vi "iWorx - Conductivity.vi"() -> ()   [LabVIEW 2012]
uses:
  vi.lib/iWorx/iWorx Set Points.ctl
  <vilib>/DAQmx/read.llb/DAQmx Read (Analog 1D Wfm NChan 1Samp).vi
  <vilib>/DAQmx/create/channels.llb/DAQmx Create Channel (AI-Voltage-Basic).vi
  <vilib>/DAQmx/miscellaneous.llb/DAQmx Fill In Error Info.vi
panel:
  in  "Reset Scale":bool
  in  "Stop":bool
  in  "Log Info Button":bool
  in  "Reset Default Cal":bool
  in  "Set Points":T1={"SP1 Voltage"=0.2, "SP1 Value"=20.0, "SP2 Voltage"=2.0, "SP2 Value"=200.0} {"SP2 Value" format="%.1f mS"; "SP2 Voltage" format="%.1f V"; "SP1 Value" format="%.1f mS"; "SP1 Voltage" format="%.1f V"}
  in  "Set Up":bool
  out "Offset(b)":dbl=-1.1111111111111112
  out "Slope(m)":dbl=5.277777777777778
  in  "Channel":u16(ring) items=["Channel 1", "Channel 2"]
  in  "Pause Button":bool
  in  "Snapshot":bool
  out "Processed Signal":dbl(knob) caption="Conductivity" scale=0.0..20.0
  out "Waveform Chart":waveform(dbl)(graph)
  in  "Sample Timing":u16(ring)=200 items=["20Hz"=50, "5 Hz"=200, "2 Hz"=500, "1 Hz"=1000, ".5 Hz"=2000, ".2 Hz"=5000]
  in  "Clear Chart":bool
  in  "Open Log":bool
  in  "Autoscale Y":bool
  out "Raw Signal":dbl(knob) scale=-10.0..10.0
  # "iWorx - Conductivity Probe - Data Logger"
  # "Sensor Input"
  # "(              ,              )"
  # "(              ,              )"
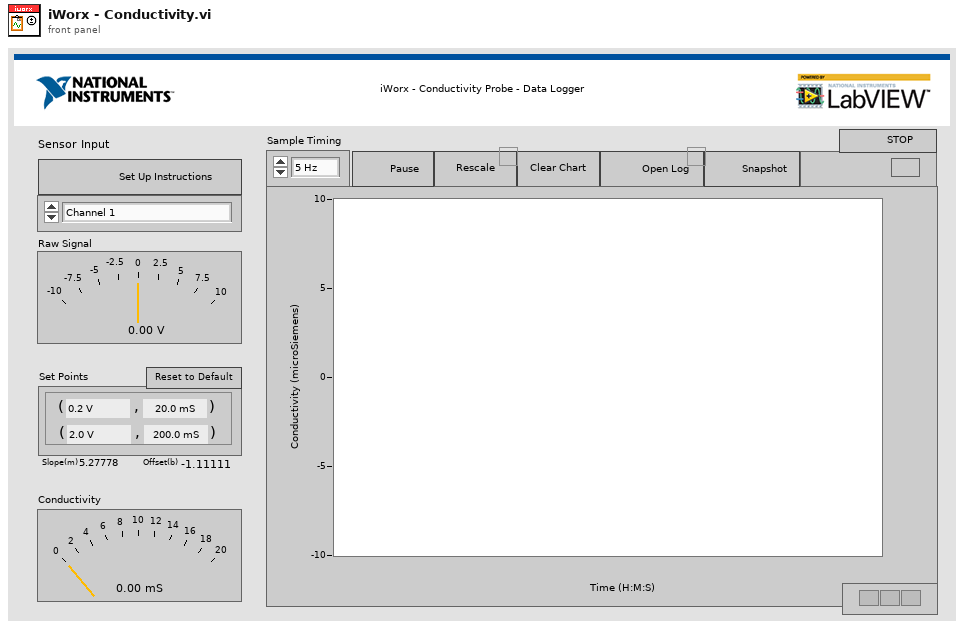
[diagram p1: front panel]
types:
  T1 = typedef "iWorx Set Points.ctl" = cluster{"SP1 Voltage":dbl, "SP1 Value":dbl, "SP2 Voltage":dbl, "SP2 Value":dbl}
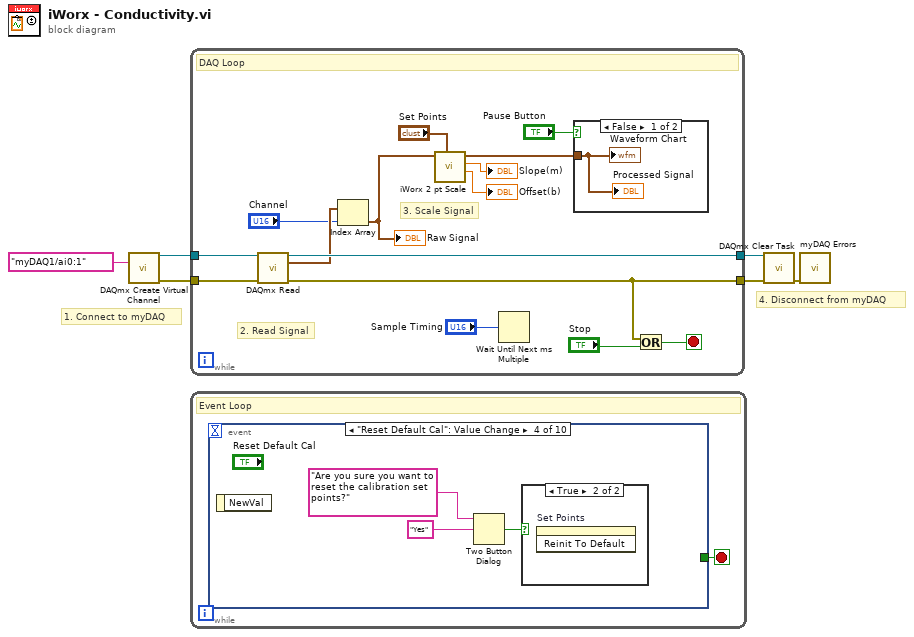
[diagram p0: block diagram]
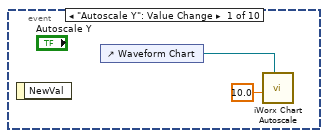
[diagram p2: hidden frame]
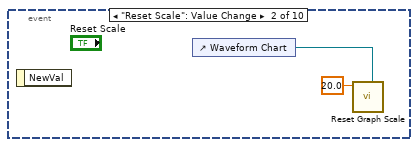
[diagram p3: hidden frame]
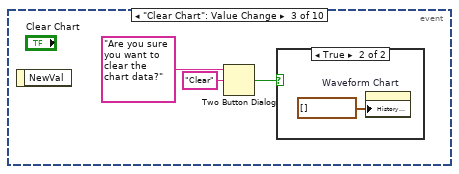
[diagram p4: hidden frame]
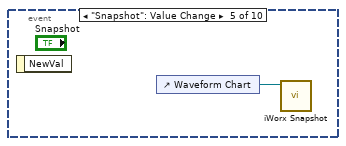
[diagram p7: hidden frame]
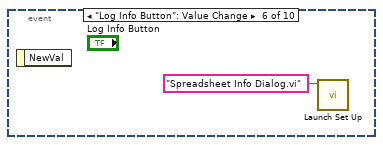
[diagram p8: hidden frame]
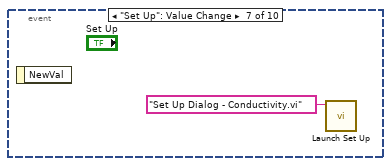
[diagram p9: hidden frame]
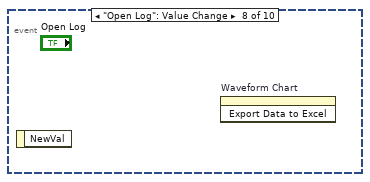
[diagram p10: hidden frame]
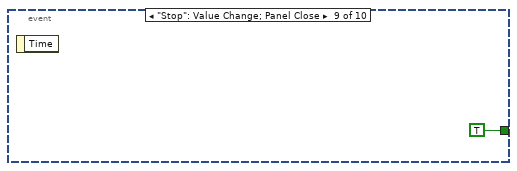
[diagram p11: hidden frame]
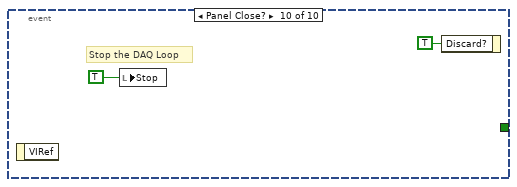
[diagram p12: hidden frame]
diagram:
  # "4. Disconnect from myDAQ"
  # "1. Connect to myDAQ"
  n1 = call-poly <vilib>:"DAQmx Create Virtual Channel.vi"("physical channels"=tag "myDAQ1/ai0:1") -> ("task out"=w3:refnum<k21>, "error out"=w2:errorcluster)  [unwired: 13 in]
  n2 = while {
    tunnel: w3 -> [w20]
    tunnel: [w19] -> w6
    tunnel: w2 -> [w18]
    tunnel: [w16] -> w5
    stop <- w17 stop-if-true
    # "3. Scale Signal"
    # "2. Read Signal"
    # "DAQ Loop"
    n3 = call-poly <vilib>:"DAQmx Read.vi"("task/channels in"=w20, "error in"=w18) -> ("task out"=w19:refnum<k21>, "data"=w14:waveform(dbl)[], "error out"=w16:errorcluster)  [unwired: 11 in]
    n4 = Index Array(array=w14, index="Channel") -> (element=w12:waveform(dbl))
    "Raw Signal" <- w12
    n5 = call "iWorx 2 pt Scale.vi"("Set Points"="Set Points", "Raw Waveform"=w12) -> ("Offset"=→"Offset(b)":dbl, "Slope"=→"Slope(m)":dbl, "Scaled Value"=w13:waveform(dbl))  [unwired: 7 in]
    n6 = Wait Until Next ms Multiple(millisecond multiple="Sample Timing") -> ()  [unwired: 1 out]
    n7 = case shown="False" "Pause Button" {
      tunnel: w13 -> [w22 _]
      frame False {
        "Waveform Chart" <- w22
        "Processed Signal" <- w22
      }
      frame True {
        # "Do Not update controls"
      }
    }
    n8 = Or(x=w16, y="Stop") -> (x .or. y?=w17:bool)
  }
  n9 = while {
    stop <- w23 stop-if-true
    # "Event Loop"
    n10 = event shown="[3] \"Reset Default Cal\": Value Change" {
      selector: _ -> [_ _ _ _ _ _ _ _ _ _]
      dyn-events: _ -> [_ _ _ _ _ _ _ _ _ _]
      timeout: _ -> [_ _ _ _ _ _ _ _ _ _]
      tunnel: [_ _ _ _ _ _ _ _ TRUE _] -> w23
      event "Autoscale Y": Value Change {
        n11 = event-data() -> ()  [unwired: 1 in, 1 out]
        n12 = control-ref of="Waveform Chart"() -> (w25:refnum<vi>)
        n13 = call "iWorx Chart Autoscale.vi"("Selection Chart"=w25, "Rounding Multiple (1)"=10.0) -> ()  [unwired: 7 in, 3 out]
      }
      event "Reset Scale": Value Change {
        n14 = event-data() -> ()  [unwired: 1 in, 1 out]
        n15 = control-ref of="Waveform Chart"() -> (w27:refnum<vi>)
        n16 = call "Reset Graph Scale.vi"("WaveformChart in"=w27, "Maximum (100)"=20.0) -> ()  [unwired: 10 in]
      }
      event "Clear Chart": Value Change {
        n17 = event-data() -> ()  [unwired: 1 in, 1 out]
        n18 = Two Button Dialog(message="Are you sure you want to clear the chart data?", 2:"Clear" ("T button name (\"OK\")")) -> (T button?=w29:bool)  [unwired: 1 in]
        n19 = case shown="True" w29 {
          frame False {
          }
          frame True {
            n20 = property on="Waveform Chart" class="WFChart (strict)"("History Data"=waveform(dbl)[] []) -> ()  [unwired: 2 in, 2 out]
          }
        }
      }
      event "Reset Default Cal": Value Change {
        n21 = event-data() -> ()  [unwired: 1 in, 1 out]
        n22 = Two Button Dialog(message="Are you sure you want to reset the calibration set points?", 2:"Yes" ("T button name (\"OK\")")) -> (T button?=w34:bool)  [unwired: 1 in]
        n23 = case shown="True" w34 {
          frame False {
          }
          frame True {
            n24 = invoke on="Set Points" class="Clust (strict)" method="Reinit To Default"() -> ()  [unwired: 3 in, 3 out]
          }
        }
      }
      event "Snapshot": Value Change {
        n25 = event-data() -> ()  [unwired: 1 in, 1 out]
        n26 = control-ref of="Waveform Chart"() -> (w35:refnum<vi>)
        n27 = call "iWorx Snapshot.vi"("WaveformChart in"=w35) -> ()  [unwired: 10 in, 1 out]
      }
      event "Log Info Button": Value Change {
        n28 = event-data() -> ()  [unwired: 1 in, 1 out]
        n29 = call "Launch Set Up.vi"("name or relative path"="Spreadsheet Info Dialog.vi") -> ()  [unwired: 9 in, 2 out]
      }
      event "Set Up": Value Change {
        n30 = event-data() -> ()  [unwired: 1 in, 1 out]
        n31 = call "Launch Set Up.vi"("name or relative path"="Set Up Dialog - Conductivity.vi") -> ()  [unwired: 9 in, 2 out]
      }
      event "Open Log": Value Change {
        n32 = event-data() -> ()  [unwired: 1 in, 1 out]
        n33 = invoke on="Waveform Chart" class="WFChart (strict)" method="Export Data to Excel"() -> ()  [unwired: 3 in, 3 out]
      }
      event "Stop": Value Change; Panel Close {
        n34 = event-data() -> ()  [unwired: 1 in, 1 out]
      }
      event Panel Close? {
        # "Stop the DAQ Loop"
        n35 = event-data() -> ()  [unwired: 1 in, 1 out]
        n36 = local write "Stop"(TRUE ("stop")) -> ()
        n37 = event-data("Discard?"=TRUE) -> ()  [unwired: 1 in, 1 out]
      }
    }
  }
  n38 = call <vilib>:"DAQmx Clear Task.vi"("task in"=w6, "error in"=w5) -> ("error out"=w1:errorcluster)  [unwired: 13 in]
  n39 = call "myDAQ Errors.vi"("error in (no error)"=w1) -> ()  [unwired: 11 in]
